vi "ScanBoxAGetSN.vi"(11 "YTESTER测试数据":T1 caption="不要修改！") -> (3 "YTESTER结论":T2)   [LabVIEW 2017]
doc: "VIDescription=取出异步扫码框A中的SN，注意要配合“异步扫码框A”使用！"
uses:
  YtCommon.lvlibp/yt`Step StepBaseInput.ctl
  YtCommon.lvlibp/yt`Step StepResult.ctl
  YtCommon.lvlibp/yt`Step TestData.ctl
  YtCommon.lvlibp/yt`Step System Queue.ctl
  Step`s VIs/YYLLGeneric/variable_W.ctl
  YtCommon.lvlibp/yt`Data-Ytester Type Data.ctl
  Step`s VIs/Step`s VIs Global.vi
  YtCommon.lvlibp
panel:
  in  "YTESTER开放参数":T4={"YTESTER_BaseInput"={"isTest"=TRUE, "isSkip"=FALSE, "StepName"="扫码框A.取出SN", "OnPass"=enum."Next", "OnFail"=enum."Terminate", "ReTestNumber"=0.0}, "取走哪个SN"=0, "赋为主SN（YTESTER测试数据）"=FALSE, "提取SN到变量(自定义建议#开头)"="不到变量"}
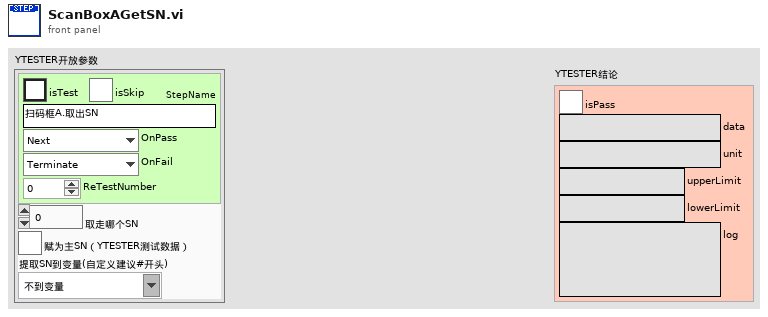
[diagram p1: front panel]
types:
  T1 = typedef "YtCommon.lvlibp/yt`Step TestData.ctl" = cluster{"Socket(From1)":i32, "SN":refnum<notifier>, "StopFlagRef":refnum<notifier>, "YT System Queue":refnum<queue>}
  T2 = typedef "YtCommon.lvlibp/yt`Step StepResult.ctl" = cluster{"isPass":bool, "data":string, "unit":string, "upperLimit":string, "lowerLimit":string, "log":string}
  T3 = typedef "YtCommon.lvlibp/yt`Step StepBaseInput.ctl" = cluster{"isTest":bool, "isSkip":bool, "StepName":string, "OnPass":enum16{"Next", "ToOVER", "Terminate"}, "OnFail":enum16{"Next", "ToOVER", "Terminate"}, "ReTestNumber":dbl}
  T4 = cluster{"YTESTER_BaseInput":T3, "取走哪个SN":u32, "赋为主SN（YTESTER测试数据）":bool, "提取SN到变量(自定义建议#开头)":string}
  T5 = typedef "variable_W.ctl" = cluster{"YT_TYPE":T6, "TypeData":string[], "Tips":string}
  T6 = typedef "YtCommon.lvlibp/yt`Data-Ytester Type Data.ctl" = enum16{"NULL", "NUM", "BOOL", "TXT", "ENUM", "TIME", "PATH", "VISA", "COMBO", "ColorBox", "RadioBtn", "Array_NUM", "Array_BOOL", "Array_TXT", "Array_ENUM", "Array_PATH", "Array_COMBO"}
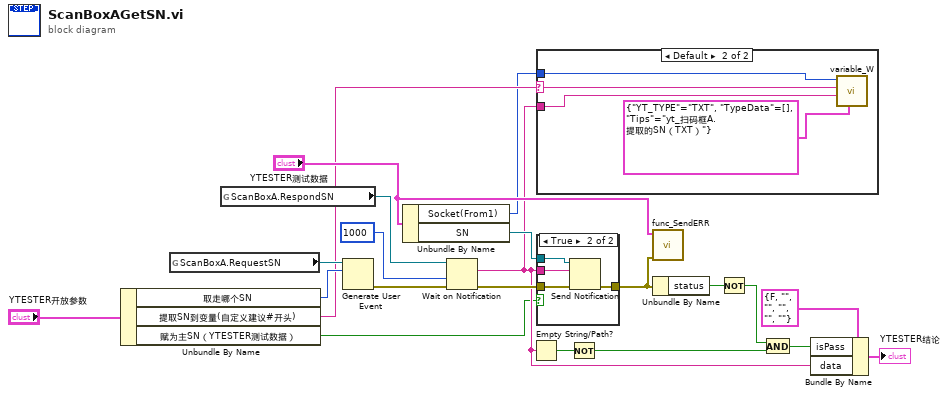
[diagram p0: block diagram]
diagram:
  n1 = Unbundle By Name("YTESTER开放参数") -> ("取走哪个SN"=w10:u32, "提取SN到变量(自定义建议#开头)"=w4:string, "赋为主SN（YTESTER测试数据）"=w1:bool)
  n2 = global read "Step`s VIs Global.vi" "ScanBoxA.RequestSN"() -> (w11:refnum<user-event>)
  n3 = global read "Step`s VIs Global.vi" "ScanBoxA.RespondSN"() -> (w9:refnum<notifier>)
  n4 = Generate User Event(user event=w11, event data cluster=w10) -> (error out=w7:errorcluster)  [unwired: 2 in, 1 out]
  n5 = Unbundle By Name("YTESTER测试数据") -> ("Socket(From1)"=w3:i32, "SN"=w18:refnum<notifier>)
  n6 = Wait on Notification(notifier=w9, timeout in ms (-1)=1000, error in (no error)=w7) -> (notification=w5:string, error out=w6:errorcluster)  [unwired: 1 in, 2 out]
  n7 = Empty String/Path?(string/path=w5) -> (empty?=w17:bool)
  n8 = case shown="Default" w4 {
    selector: w4 -> [_ w24]
    tunnel: w3 -> [_ w25]
    tunnel: w5 -> [_ w23]
    frame "不到变量" {
    }
    frame Default {
      n9 = call "variable_W.vi"("附加的Information"=T5 {"YT_TYPE"=enum."TXT", "TypeData"=[], "Tips"="yt_扫码框A.提取的SN（TXT）"}, "待写入池的输入控件"=w23, "待写入池变量名称"=w24, "函数池名称 in"=w25) -> ()  [unwired: 5 in, 3 out]
    }
  }
  n10 = case shown="True" w1 {
    tunnel: w18 -> [_ w30]
    tunnel: w6 -> [w26 w29]
    tunnel: w5 -> [_ w28]
    tunnel: [w26 w27] -> w2
    frame False {
    }
    frame True {
      n11 = Send Notification(notification=w28, notifier=w30, error in (no error)=w29) -> (error out=w27:errorcluster)  [unwired: 1 out]
    }
  }
  n12 = Not(x=w17) -> (.not. x?=w16:bool)
  n13 = call "func_SendERR.vi"("ERR (String\\Errclust)"=w2, "YTESTER测试数据 in"="YTESTER测试数据") -> ()  [unwired: 9 in, 1 out]
  n14 = Unbundle By Name(w2) -> ("status"=w14:bool)
  n15 = Not(x=w14) -> (.not. x?=w12:bool)
  n16 = And(x=w12, y=w16) -> (x .and. y?=w13:bool)
  n17 = Bundle By Name(cluster=T2 {"isPass"=FALSE, "data"="", "unit"="", "upperLimit"="", "lowerLimit"="", "log"=""} ("Result"), "isPass"=w13, "data"=w5) -> (→"YTESTER结论":T2)
